vi "save channels to stacked multi-tiff files.vi"(8 "frame number in":i32, 9 "last frame":bool, 11 "image data in":dbl[][](array[numeric])) -> ()   [LabVIEW 2012]
doc: "SciScan 1.2 160622"
uses:
  Custom Controls/file format type def.ctl
  GFG/GFGpathGet.vi
  GFG/GFGnumericGet.vi
  GFG/GFGstringGet.vi
  Libtiff3/libtiff3.llb/libtiff3.lvlib
  GFG/GFG library.lvlib
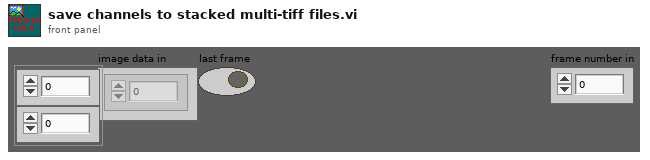
[diagram p1: front panel]
types:
  T1 = typedef "file format type def.ctl" = enum16{"16bit raw", "32bit raw", "16bit multi-tiff (interleave)", "16bit multi-tiff (separate)", "16bit multi-tiff (stacked)", "32bit multi-tiff (interleave)", "32bit multi-tiff (separate)", "32bit multi-tiff (stacked)", "16bit tiff series (interleave)", "16bit tiff series (separate)", "16bit tiff series (stacked)", "32bit tiff series (interleave)", "32bit tiff series (separate)", "32bit tiff series (stacked)"}
  T2 = cluster{"no..of.frames.to.acquire":dbl, "x.pixels":dbl, "y.pixels":dbl, "x.pixel.sz":dbl, "y.pixel.sz":dbl}
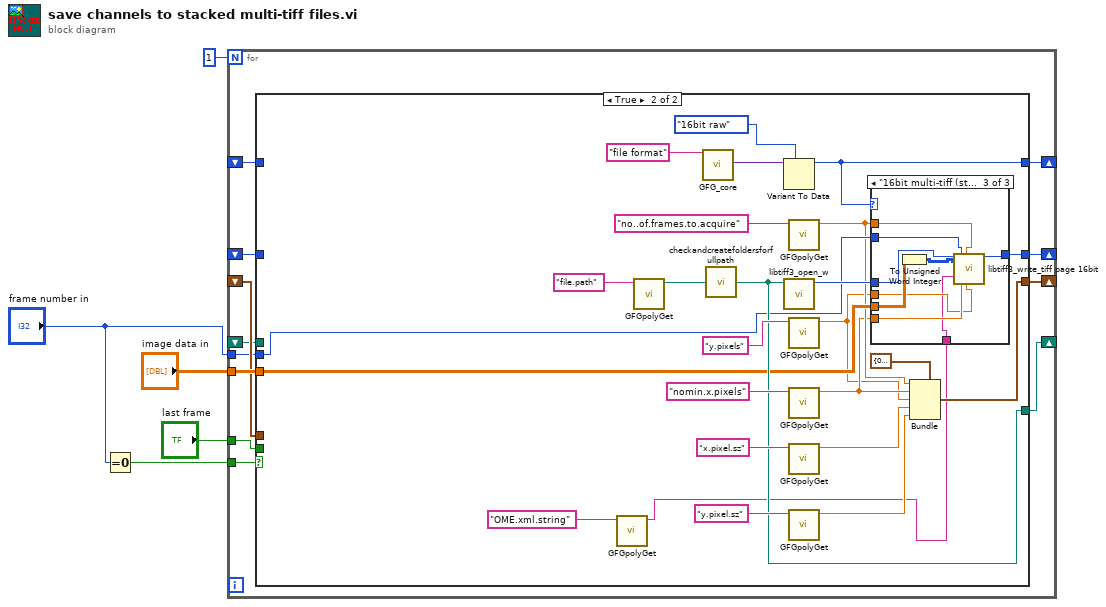
[diagram p0: block diagram]
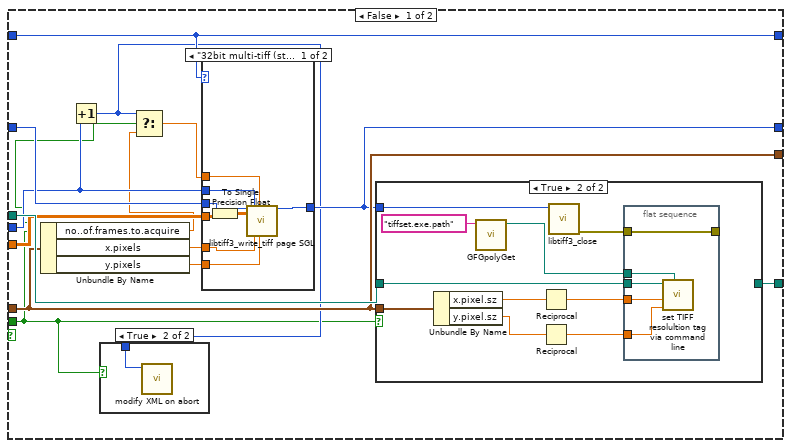
[diagram p2: hidden frame]
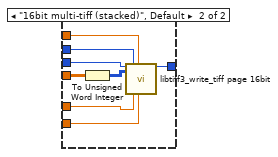
[diagram p4: hidden frame]
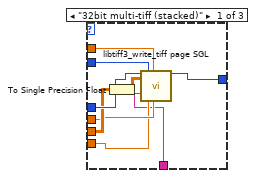
[diagram p6: hidden frame]
diagram:
  n1 = Equal To 0?(x="frame number in") -> (x = 0?=w4:bool)
  n2 = for {
    N: 1 -> [_]
    tunnel: w4 -> [w17]
    shift-right: [w16] -> _
    shift-left: _ -> [w15]
    tunnel: "image data in" -> [w14]
    shift-right: [w13] -> _
    shift-left: _ -> [w12]
    shift-right: [w11] -> _
    shift-left: _ -> [w10]
    shift-right: [w9] -> _
    shift-left: _ -> [w8]
    tunnel: "last frame" -> [w7]
    tunnel: "frame number in" -> [w6]
    n3 = case shown="True" w17 {
      tunnel: w12 -> [w25 _]
      tunnel: [w23 w69] -> w16
      tunnel: w15 -> [w29 _]
      tunnel: w14 -> [w30 w73]
      tunnel: [w25 w74] -> w13
      tunnel: [w24 w77] -> w11
      tunnel: w10 -> [w24 _]
      tunnel: [w28 w76] -> w9
      tunnel: w8 -> [w31 _]
      tunnel: w7 -> [w18 _]
      tunnel: w6 -> [w22 w71]
      frame False {
        n4 = Unbundle By Name(w24) -> ("no..of.frames.to.acquire"=w21:dbl, "x.pixels"=w27:dbl, "y.pixels"=w26:dbl)
        n5 = Increment(x=w22) -> (x+1=w19:i32)
        n6 = case shown="True" w18 {
          tunnel: w19 -> [_ w32]
          frame False {
          }
          frame True {
            n7 = call "modify XML on abort.vi"("frame number"=w32) -> ()  [unwired: 10 in, 1 out]
          }
        }
        n8 = Select(t=w19, s=w18, f=w21) -> (s? t:f=w20:dbl)
        n9 = case shown="\"32bit multi-tiff (stacked)\"" w25 {
          tunnel: w30 -> [w36 w48]
          tunnel: w29 -> [w40 w46]
          tunnel: [w37 w45] -> w23
          tunnel: w20 -> [w38 w44]
          tunnel: w22 -> [w39 w43]
          tunnel: w27 -> [w35 w42]
          tunnel: w26 -> [w34 w41]
          frame "32bit multi-tiff (stacked)" {
            n10 = To Single Precision Float(number=w36) -> (single precision float=w33:sgl[][])
            n11 = call "libtiff3_write_tiff page SGL.vi"("Handle"=w40, "Image Pixels (Float)"=w33, "page"=w39, "x.pixels"=w35, "totalpages"=w38, "y.pixels"=w34) -> ("Handle out"=w37:i32)  [unwired: 12 in, 1 out]
          }
          frame "16bit multi-tiff (stacked)", Default {
            n12 = To Unsigned Word Integer(number=w48) -> (unsigned 16bit integer=w47:u16[][])
            n13 = call "libtiff3_write_tiff page 16bit.vi"("Handle"=w46, "Image Pixels (U16)"=w47, "page"=w43, "x.pixels"=w42, "totalpages"=w44, "y.pixels"=w41) -> ("Handle out"=w45:i32)  [unwired: 12 in, 1 out]
          }
        }
        n14 = case shown="True" w18 {
          tunnel: w24 -> [_ w54]
          tunnel: w31 -> [w49 w53]
          tunnel: w23 -> [_ w52]
          tunnel: [w49 _] -> w28
          frame False {
          }
          frame True {
            n15 = Unbundle By Name(w54) -> ("x.pixel.sz"=w55:dbl, "y.pixel.sz"=w56:dbl)
            n16 = call-poly "GFGpolyGet.vi"("Variable Name in"="tiffset.exe.path") -> ("Path"=w50:path)  [unwired: 8 in, 2 out]
            n17 = Reciprocal(x=w55) -> (1/x=w57:dbl)
            n18 = Reciprocal(x=w56) -> (1/x=w58:dbl)
            n19 = call "libtiff3_close.vi"("Handle"=w52) -> ("error out"=w59:errorcluster)  [unwired: 9 in]
            n20 = flat-sequence {
              tunnel: w53 -> [w64]
              tunnel: w59 -> [w61]
              tunnel: w57 -> [w63]
              tunnel: w58 -> [w62]
              tunnel: [w61] -> _
              tunnel: w50 -> [w60]
              frame #0 {
                n21 = call "set TIFF resolultion tag via command line.vi"("tiffset.exe file path"=w60, "y pixels per m"=w62, "x pixels per m"=w63, "TIFF file path"=w64) -> ()  [unwired: 8 in]
              }
            }
          }
        }
      }
      frame True {
        n22 = call-poly "GFGpolyGet.vi"("Variable Name in"="OME.xml.string" ("Tag in")) -> ("String"=w65:string)  [unwired: 9 in, 1 out]
        n23 = call-poly "GFGpolyGet.vi"("Variable Name in"="file.path") -> ("Path"=w75:path)  [unwired: 8 in, 2 out]
        n24 = call "GFG_core.vi"("Variable Name in"="file format") -> ("Variant Out"=w88:variant)  [unwired: 12 in, 6 out]
        n25 = call "checkandcreatefoldersforfullpath.vi"("Path IN"=w75) -> ("Path OUT"=w76:path)  [unwired: 4 in]
        n26 = Variant To Data(type=file_format_type_def."16bit raw" ("file format"), Variant=w88) -> (data=w74:T1)  [unwired: 1 in, 1 out]
        n27 = call "libtiff3_open_w.vi"("Input path"=w76) -> ("handle"=w72:i32)  [unwired: 9 in, 1 out]
        n28 = call-poly "GFGpolyGet.vi"("Variable Name in"="no..of.frames.to.acquire") -> ("Numeric"=w70:dbl)  [unwired: 8 in, 2 out]
        n29 = call-poly "GFGpolyGet.vi"("Variable Name in"="y.pixels" ("Tag in")) -> ("Numeric"=w67:dbl)  [unwired: 8 in, 2 out]
        n30 = call-poly "GFGpolyGet.vi"("Variable Name in"="nomin.x.pixels" ("Tag in")) -> ("Numeric"=w68:dbl)  [unwired: 8 in, 2 out]
        n31 = call-poly "GFGpolyGet.vi"("Variable Name in"="x.pixel.sz" ("Tag in")) -> ("Numeric"=w80:dbl)  [unwired: 8 in, 2 out]
        n32 = call-poly "GFGpolyGet.vi"("Variable Name in"="y.pixel.sz" ("Tag in")) -> ("Numeric"=w79:dbl)  [unwired: 8 in, 2 out]
        n33 = case shown="\"16bit multi-tiff (stacked)\"" w74 {
          tunnel: w73 -> [w94 _ w105]
          tunnel: w72 -> [w95 w99 w106]
          tunnel: w71 -> [w96 _ w107]
          tunnel: w70 -> [w97 _ w108]
          tunnel: [w98 w99 w101] -> w69
          tunnel: w68 -> [w91 _ w103]
          tunnel: w67 -> [w92 _ w102]
          tunnel: w65 -> [w90 _ w100]
          frame "32bit multi-tiff (stacked)" {
            n34 = To Single Precision Float(number=w94) -> (single precision float=w93:sgl[][])
            n35 = call "libtiff3_write_tiff page SGL.vi"("Handle"=w95, "Image Pixels (Float)"=w93, "Image Description"=w90, "page"=w96, "x.pixels"=w91, "totalpages"=w97, "y.pixels"=w92) -> ("Handle out"=w98:i32)  [unwired: 11 in, 1 out]
          }
          frame Default {
          }
          frame "16bit multi-tiff (stacked)" {
            n36 = To Unsigned Word Integer(number=w105) -> (unsigned 16bit integer=w104:u16[][])
            n37 = call "libtiff3_write_tiff page 16bit.vi"("Handle"=w106, "Image Pixels (U16)"=w104, "ImageDescription"=w100, "page"=w107, "x.pixels"=w103, "totalpages"=w108, "y.pixels"=w102) -> ("Handle out"=w101:i32)  [unwired: 11 in, 1 out]
          }
        }
        n38 = Bundle(cluster=T2 {"no..of.frames.to.acquire"=0.0, "x.pixels"=0.0, "y.pixels"=0.0, "x.pixel.sz"=0.0, "y.pixel.sz"=0.0} ("output cluster"), "no..of.frames.to.acquire"=w70, "x.pixels"=w68, "y.pixels"=w67, "x.pixel.sz"=w80, "y.pixel.sz"=w79) -> (w77:T2)
      }
    }
  }
